vi "Actor API Type.vi"(11 "Test 1 in":refnum<class "Test Caller.lvclass">) -> (2 "Actor API Type":refnum<class "Actor API.lvclass">)   [LabVIEW 2022 SP3, in "Scratchpad.lvlib" / "Test Caller.lvlib" / "Test Caller.lvclass"]
uses:
  Test Caller.lvclass
  Test Caller.lvclass/Test Caller.ctl
  Test Caller API/Test Caller API.lvclass
  C:/dev/lv/2022/lv-artifex/Artifex/Actor Proxy/Actor API.lvclass
  C:/dev/lv/2022/lv-artifex/Scratchpad/Test Caller/Test 1 API/Test Caller API.lvclass
  Artifex/Actor Proxy/Actor API.lvclass
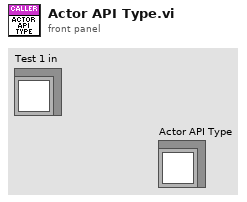
[diagram p1: front panel]
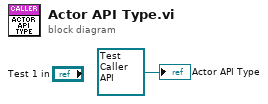
[diagram p0: block diagram]
diagram:
  "Actor API Type" <- refnum<class "Test Caller API.lvclass"> refnum ("Scratchpad.lvlib:Test 1.lvlib:Test 1 API.lvclass")
